vi "Find STL Path.vi"(8 "Error In":errorcluster) -> (0 "Error Out":errorcluster, 2 "Array for myRoboLab Parts":T1(array[cluster]))   [LabVIEW 2020]
doc: "This VI adds to all the STL files the path to programatically find them wherever the project is saved."
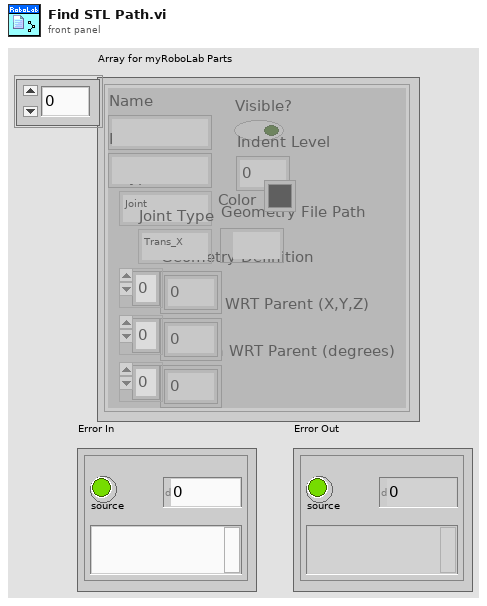
[diagram p1: front panel]
types:
  T1 = cluster{"Name":string, "Parent":string, "Type":enum16{"Joint", "Box", "Cylinder", "Cone", "Sphere", "ASE File", "VRML File", "STL File", "Space"}, "Visible?":bool, "Geometry Definition":dbl[], "Position WRT Parent (X,Y,Z)":dbl[], "Rotation WRT Parent (degrees)":dbl[], "Joint Type":enum16{"Trans_X", "Trans_Y", "Trans_Z", "Rot_X", "Rot_Y", "Rot_Z", "None"}, "Geometry File Path":path, "Indent Level":i32, "Color":u32}[]
  T2 = cluster{"Name":string, "Parent":string, "Type":enum16{"Joint", "Box", "Cylinder", "Cone", "Sphere", "ASE File", "VRML File", "STL File", "Space"}, "Visible?":bool, "Geometry Definition":dbl[], "Position WRT Parent (X,Y,Z)":dbl[], "Rotation WRT Parent (degrees)":dbl[], "Joint Type":enum16{"Trans_X", "Trans_Y", "Trans_Z", "Rot_X", "Rot_Y", "Rot_Z", "None"}, "Geometry File Path":path, "Indent Level":i32, "Color":u32}
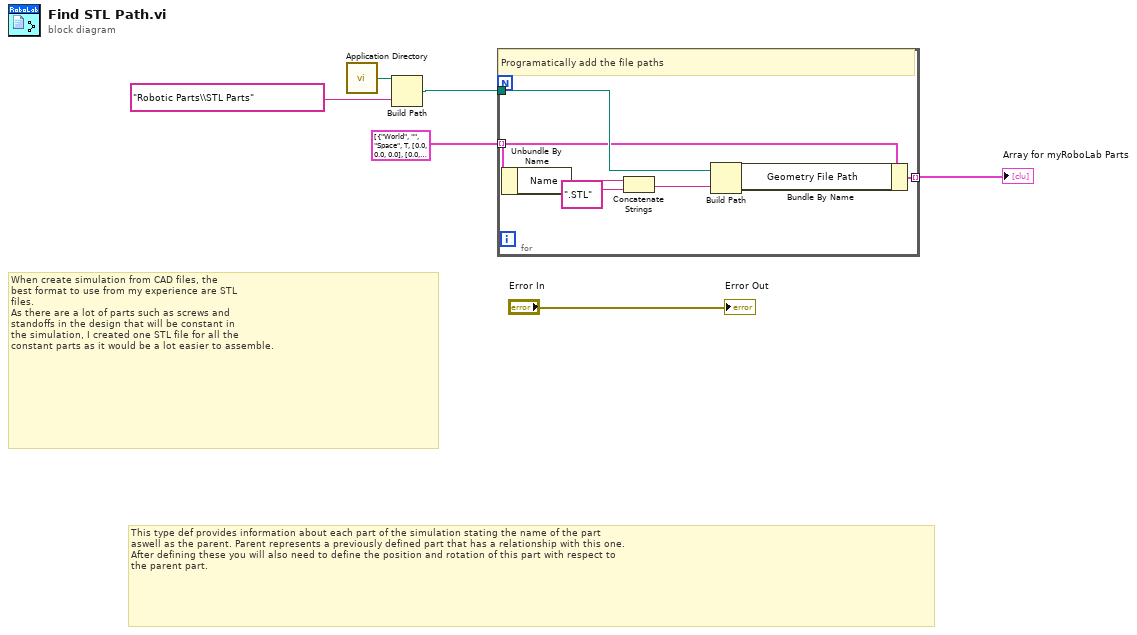
[diagram p0: block diagram]
diagram:
  # "When create simulation from CAD files, the \nbest format to use from my experience are STL\nfiles. \nAs there are a lot of parts such as screws and \nstandoffs in the design that will be constant in\nthe simulation, I created one STL file for all the \nconstant parts as it would be a lot easier to assemble."
  # "This type def provides information about each part of the simulation stating the name of the part\naswell as the parent. Parent represents a previously defined part that has a relationship with this one.\nAfter defining these you will also need to define the position and rotation of this part with respect to \nthe parent part."
  n1 = call <vilib>:"Application Directory.vi"() -> ("Application Directory"=w3:path)
  n2 = Build Path(base path=w3, name or relative path="Robotic Parts\\STL Parts") -> (appended path=w5:path)
  n3 = for {
    tunnel: T1 [{"Name"="World", "Parent"="", "Type"=enum."Space", "Visible?"=TRUE, "Geometry Definition"=[0.0, 0.0, 0.0], "Position WRT Parent (X,Y,Z)"=[0.0, 0.0, 0.0], "Rotation WRT Parent (degrees)"=[0.0, 0.0, 0.0, 0.0], "Joint Type"=enum."None", "Geometry File Path"=path "", "Indent Level"=50, "Color"=12500670}, {"Name"="Base", "Parent"="World", "Type"=enum."STL File", "Visible?"=TRUE, "Geometry Definition"=[0.0, 0.0, 0.0], "Position WRT Parent (X,Y,Z)"=[60.0, -300.0, -50.0], "Rotation WRT Parent (degrees)"=[-10.0, 40.0, -15.0, 0.0], "Joint Type"=enum."None", "Geometry File Path"=path "C:/Users/ukkanakm/Desktop/myRobo/Robotic Parts/STL Parts/Base.STL", "Indent Level"=0, "Color"=13816530}, {"Name"="Joint 1 Plate", "Parent"="Base", "Type"=enum."Cylinder", "Visible?"=TRUE, "Geometry Definition"=[5.0, 40.0, 1.0], "Position WRT Parent (X,Y,Z)"=[66.0, 207.0, 230.0], "Rotation WRT Parent (degrees)"=[0.0, 0.0, 0.0, 0.0], "Joint Type"=enum."None", "Geometry File Path"=path "", "Indent Level"=50, "Color"=13816530}, {"Name"="Joint 1", "Parent"="Joint 1 Plate", "Type"=enum."Joint", "Visible?"=TRUE, "Geometry Definition"=[1.0, 1.0, 1.0], "Position WRT Parent (X,Y,Z)"=[0.0, 0.0, 0.0], "Rotation WRT Parent (degrees)"=[0.0, 0.0, 0.0, 0.0], "Joint Type"=enum."Rot_Z", "Geometry File Path"=path "", "Indent Level"=0, "Color"=13816530}, {"Name"="Motor 1", "Parent"="Joint 1", "Type"=enum."STL File", "Visible?"=TRUE, "Geometry Definition"=[0.0, 0.0, 0.0], "Position WRT Parent (X,Y,Z)"=[-65.0, -205.0, -230.0], "Rotation WRT Parent (degrees)"=[0.0, 0.0, 0.0, 0.0], "Joint Type"=enum."None", "Geometry File Path"=path "C:/Users/ukkanakm/Desktop/myRobo/Robotic Parts/STL Parts/Motor 1.STL", "Indent Level"=0, "Color"=13816530}, {"Name"="Joint 2 Plate", "Parent"="Motor 1", "Type"=enum."Cylinder", "Visible?"=TRUE, "Geometry Definition"=[5.0, 10.0, 1.0], "Position WRT Parent (X,Y,Z)"=[-278.0, 215.0, 40.0], "Rotation WRT Parent (degrees)"=[0.0, 90.0, 4.0, 0.0], "Joint Type"=enum."None", "Geometry File Path"=path "", "Indent Level"=0, "Color"=12500670}, {"Name"="Joint 2", "Parent"="Joint 2 Plate", "Type"=enum."Joint", "Visible?"=TRUE, "Geometry Definition"=[1.0, 1.0, 1.0], "Position WRT Parent (X,Y,Z)"=[0.0, 0.0, 0.0], "Rotation WRT Parent (degrees)"=[0.0, 0.0, 0.0, 0.0], "Joint Type"=enum."Rot_Z", "Geometry File Path"=path "", "Indent Level"=0, "Color"=13816530}, {"Name"="Motor 2", "Parent"="Joint 2", "Type"=enum."STL File", "Visible?"=TRUE, "Geometry Definition"=[0.0, 0.0, 0.0], "Position WRT Parent (X,Y,Z)"=[-95.0, -210.0, -280.0], "Rotation WRT Parent (degrees)"=[0.0, 92.0, 3.0, 0.0], "Joint Type"=enum."None", "Geometry File Path"=path "C:/Users/ukkanakm/Desktop/myRobo/Robotic Parts/STL Parts/Motor 2.STL", "Indent Level"=0, "Color"=13816530}, {"Name"="Joint 3 Plate", "Parent"="Motor 2", "Type"=enum."Cylinder", "Visible?"=TRUE, "Geometry Definition"=[5.0, 10.0, 1.0], "Position WRT Parent (X,Y,Z)"=[-395.0, 230.0, 35.0], "Rotation WRT Parent (degrees)"=[0.0, 90.0, 5.0, 0.0], "Joint Type"=enum."Trans_X", "Geometry File Path"=path "", "Indent Level"=0, "Color"=12500670}, {"Name"="Joint 3", "Parent"="Joint 3 Plate", "Type"=enum."Joint", "Visible?"=TRUE, "Geometry Definition"=[1.0, 1.0, 1.0], "Position WRT Parent (X,Y,Z)"=[0.0, 0.0, 0.0], "Rotation WRT Parent (degrees)"=[0.0, 0.0, 0.0, 0.0], "Joint Type"=enum."Rot_Z", "Geometry File Path"=path "", "Indent Level"=0, "Color"=0}, {"Name"="Motor 3", "Parent"="Joint 3", "Type"=enum."STL File", "Visible?"=TRUE, "Geometry Definition"=[0.0, 0.0, 0.0], "Position WRT Parent (X,Y,Z)"=[-90.0, -220.0, -400.0], "Rotation WRT Parent (degrees)"=[0.0, 95.0, -15.0, 0.0], "Joint Type"=enum."None", "Geometry File Path"=path "C:/Users/ukkanakm/Desktop/myRobo/Robotic Parts/STL Parts/Motor 3.STL", "Indent Level"=0, "Color"=13816530}] -> [w8] mode=indexing
    tunnel: w5 -> [w10]
    tunnel: [w7] -> w6 mode=indexing
    # "Programatically add the file paths"
    n4 = Unbundle By Name(w8) -> ("Name"=w13:string)
    n5 = Concatenate Strings(w13, ".STL" ("string")) -> (w11:string)
    n6 = Build Path(base path=w10, name or relative path=w11) -> (appended path=w9:path)
    n7 = Bundle By Name(cluster=w8, "Geometry File Path"=w9) -> (w7:T2)
  }
  "Array for myRoboLab Parts" <- w6
  "Error Out" <- "Error In"
